vi "DimIndicators.dispatcher.vi"(9 "stop":refnum<k4>) -> ()   [LabVIEW 2014, in "DimIndicators.lvlib"]
doc: "Dispatcher of service data for the DimIndicators library. By default, this is started by the dim_operate method of the LVDimInterface library."
uses:
  DimIndicators.lvlib
  DimIndicators.numericType.ctl
  DimIndicators.numericArrayType.ctl
  DimIndicators.anyType.ctl
  DimIndicators.actionType.ctl
  LVDimInterface/LVDimInterface.lvlib
panel:
  in  "anyType":T1
  in  "numericArray":T2
  out "Numeric":i32
  in  "numericType":T3
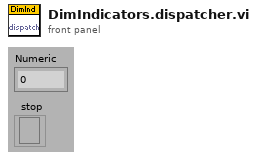
[diagram p1: front panel]
types:
  T1 = typedef "DimIndicators.lvlib/DimIndicators.anyType.ctl" = cluster{"data":string, "no link":bool, "quality":i32, "timeStamp":dbl}
  T2 = typedef "DimIndicators.lvlib/DimIndicators.numericArrayType.ctl" = cluster{"data":dbl[], "no link":bool, "quality":i32, "timeStamp":dbl}
  T3 = typedef "DimIndicators.lvlib/DimIndicators.numericType.ctl" = cluster{"data":dbl, "no link":bool, "quality":i32, "timeStamp":dbl}
  T4 = typedef "DimIndicators.lvlib/DimIndicators.actionType.ctl" = enum16{"dic_info_service", "dic_release_service", "init", "getControlRef", "getCallbackID", "close"}
  T5 = typedef "DimIndicators.lvlib/DimIndicators.dataType.ctl" = enum16{"unknown", "numeric", "numericArray", "any"}
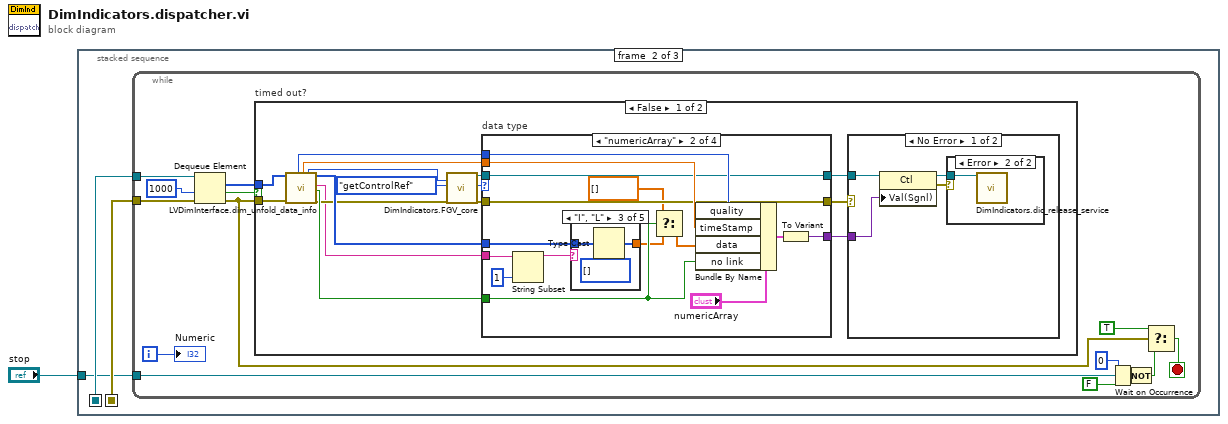
[diagram p0: block diagram]
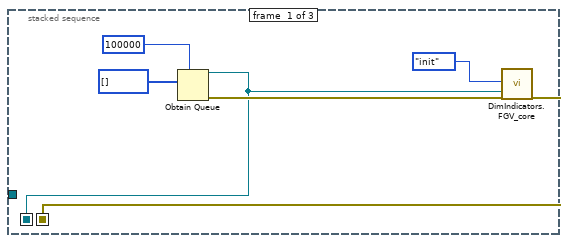
[diagram p2: hidden frame]
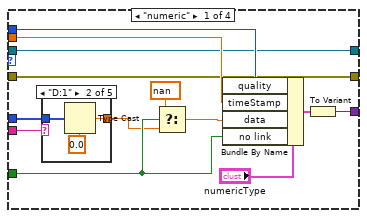
[diagram p5: hidden frame]
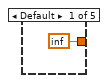
[diagram p6: hidden frame]
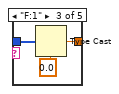
[diagram p7: hidden frame]
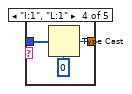
[diagram p8: hidden frame]
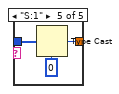
[diagram p9: hidden frame]
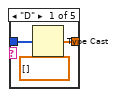
[diagram p10: hidden frame]
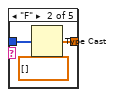
[diagram p11: hidden frame]
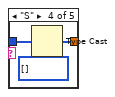
[diagram p12: hidden frame]
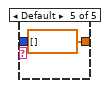
[diagram p13: hidden frame]
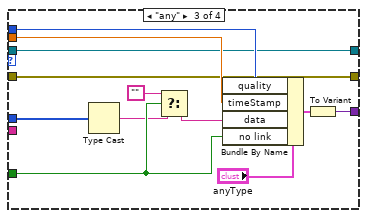
[diagram p14: hidden frame]
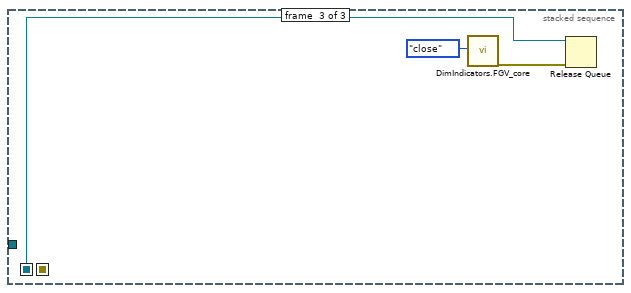
[diagram p17: hidden frame]
diagram:
  n1 = stacked-sequence {
    seq-local: [w4 _ _] -> [_ w9 _]
    seq-local: [w3 _ _] -> [_ w10 w115]
    tunnel: "stop" -> [_ w8 _]
    frame #0 {
      n2 = Obtain Queue(max queue size (-1, unlimited)=100000, element data type=i8[] []) -> (queue out=w3:refnum<queue>, error out=w5:errorcluster)  [unwired: 3 in, 1 out]
      n3 = call "DimIndicators.FGV_core.vi"("actions"=DimIndicators.actionType."init", "queueRef"=w3, "error in (no error)"=w5) -> ("error out"=w4:errorcluster)  [unwired: 13 in, 3 out]
    }
    frame #1 {
      n4 = while {
        tunnel: w10 -> [w24]
        tunnel: w9 -> [w20]
        tunnel: w8 -> [w13]
        i -> [w16]
        stop <- w22 stop-if-true
        n5 = Dequeue Element(queue=w24, timeout in ms (-1)=1000, error in (no error)=w20) -> (element=w18:i8[], timed out?=w19:bool, error out=w17:errorcluster)  [unwired: 1 out]
        n6 = case "timed out?" shown="False" w19 {
          tunnel: w17 -> [w40 _]
          tunnel: w18 -> [w39 _]
          frame False {
            n7 = call "LVDimInterface.dim_unfold_data_info.vi"("rawData"=w39, "error in (no error)"=w40) -> ("quality"=w38:i32, "timeStamp"=w37:dbl, "callBackID"=w31:i32, "data"=w36:i8[], "typeDescriptor"=w28:string, "no link"=w35:bool, "error out"=w33:errorcluster)  [unwired: 7 in, 4 out]
            n8 = call "DimIndicators.FGV_core.vi"("callBackID"=w31, "actions"=DimIndicators.actionType."getControlRef", "error in (no error)"=w33) -> ("controlRef out"=w27:refnum<vi>, "dataType out"=w29:T5, "error out"=w32:errorcluster)  [unwired: 13 in, 1 out]
            n9 = case "data type" shown="\"numericArray\"" w29 {
              tunnel: w38 -> [w57 w85 w110 _]
              tunnel: w37 -> [w56 w84 w109 _]
              tunnel: w36 -> [w55 w83 w108 _]
              tunnel: w35 -> [w49 w75 w103 _]
              tunnel: [w53 w81 w106 _] -> w34
              tunnel: [w52 w80 w105 w113] -> w25
              tunnel: w32 -> [w52 w80 w105 w113]
              tunnel: w28 -> [w51 w79 _ _]
              tunnel: [w50 w76 w104 w112] -> w26
              tunnel: w27 -> [w50 w76 w104 w112]
              frame "numeric" {
                n10 = case shown="\"D:1\"" w51 {
                  tunnel: w55 -> [_ w62 w65 w68 w71]
                  tunnel: [inf ("Positive Infinity") w60 w63 w66 w69] -> w48
                  frame Default {
                  }
                  frame "D:1" {
                    n11 = Type Cast(type=0.0, x=w62) -> (*(type *) &x=w60:dbl)
                  }
                  frame "F:1" {
                    n12 = Type Cast(type=sgl 0.0, x=w65) -> (*(type *) &x=w63:sgl)
                  }
                  frame "I:1", "L:1" {
                    n13 = Type Cast(type=0, x=w68) -> (*(type *) &x=w66:i32)
                  }
                  frame "S:1" {
                    n14 = Type Cast(type=i16 0, x=w71) -> (*(type *) &x=w69:i16)
                  }
                }
                n15 = Select(t=nan, s=w49, f=w48) -> (s? t:f=w47:dbl)
                n16 = Bundle By Name(cluster="numericType", "quality"=w57, "timeStamp"=w56, "data"=w47, "no link"=w49) -> (w54:T3)
                n17 = To Variant(anything=w54) -> (Variant=w53:variant)
              }
              frame "numericArray" {
                n18 = String Subset(string=w79, length (rest)=1 ("length (rest)")) -> (substring=w77:string)  [unwired: 1 in]
                n19 = case shown="\"I\", \"L\"" w77 {
                  tunnel: w83 -> [w89 w92 w95 w98 _]
                  tunnel: [w88 w91 w94 w97 dbl[] []] -> w73
                  frame "D" {
                    n20 = Type Cast(type=dbl[] [], x=w89) -> (*(type *) &x=w88:dbl[])
                  }
                  frame "F" {
                    n21 = Type Cast(type=sgl[] [], x=w92) -> (*(type *) &x=w91:sgl[])
                  }
                  frame "I", "L" {
                    n22 = Type Cast(type=i32[] [], x=w95) -> (*(type *) &x=w94:i32[])
                  }
                  frame "S" {
                    n23 = Type Cast(type=i16[] [], x=w98) -> (*(type *) &x=w97:i16[])
                  }
                  frame Default {
                  }
                }
                n24 = Select(t=dbl[] [], s=w75, f=w73) -> (s? t:f=w74:dbl[])
                n25 = Bundle By Name(cluster="numericArray", "quality"=w85, "timeStamp"=w84, "data"=w74, "no link"=w75) -> (w82:T2)
                n26 = To Variant(anything=w82) -> (Variant=w81:variant)
              }
              frame "any" {
                n27 = Type Cast(x=w108) -> (*(type *) &x=w102:string)  [unwired: 1 in]
                n28 = Select(t="", s=w103, f=w102) -> (s? t:f=w101:string)
                n29 = Bundle By Name(cluster="anyType", "quality"=w110, "timeStamp"=w109, "data"=w101, "no link"=w103) -> (w107:T1)
                n30 = To Variant(anything=w107) -> (Variant=w106:variant)
              }
              frame Default {
              }
            }
            n31 = case shown="No Error" w25 {
              tunnel: w34 -> [w44 _]
              tunnel: w26 -> [w43 _]
              frame No Error {
                n32 = property on="Property Node" class="Ctl"(reference=w43, "Val(Sgnl)"=w44) -> (reference out=w41:refnum<vi>, error out=w42:errorcluster)  [unwired: 1 in]
                n33 = case shown="Error" w42 {
                  tunnel: w41 -> [_ w45]
                  frame No Error {
                  }
                  frame Error {
                    n34 = call "DimIndicators.dic_release_service.vi"("controlRef"=w45) -> ()  [unwired: 18 in, 1 out]
                  }
                }
              }
              frame Error {
              }
            }
          }
          frame True {
          }
        }
        n35 = Wait on Occurrence(1:FALSE ("ignore previous (T)"), 2:w13, 3:0 ("ms timeout (-1)")) -> (0:w15:bool)
        n36 = Not(x=w15) -> (.not. x?=w14:bool)
        n37 = Select(t=TRUE, s=w17, f=w14) -> (s? t:f=w22:bool)
        "Numeric" <- w16
      }
    }
    frame #2 {
      n38 = call "DimIndicators.FGV_core.vi"("actions"=DimIndicators.actionType."close") -> ("error out"=w116:errorcluster)  [unwired: 15 in, 3 out]
      n39 = Release Queue(queue=w115, error in (no error)=w116) -> ()  [unwired: 1 in, 3 out]
    }
  }
